vi "20191114_SR400 monitoring.vi"(10 "?":bool, 11 "?":bool) -> ()   [LabVIEW 2015]
uses:
  Libraries/SR400/Public/Typedefs/Counter.ctl
  Libraries/SR400/SR400.lvlib
panel:
  in  "Count Time Set":dbl[unit]=0.01
  in  "VISA resource name":refnum<visa-resource-name>="GPIB0::18::INSTR"
  out "Counts":dbl=46900.0 format="%#_6e"
  out "Count plot":dbl(graph)=46900.0
  # "Saturate @\n3E+7 c/s"
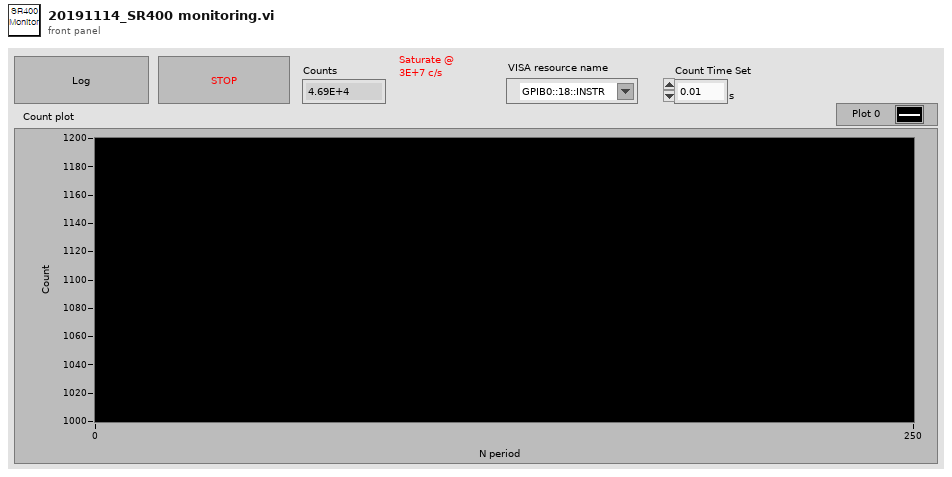
[diagram p1: front panel]
types:
  T1 = enum16{"open", "replace", "create", "open or create", "replace or create", "replace or create with confirmation"}
  T2 = typedef "SR400.lvlib/Counter.ctl" = enum16{"Counter A", "Counter B", "Counter T"}
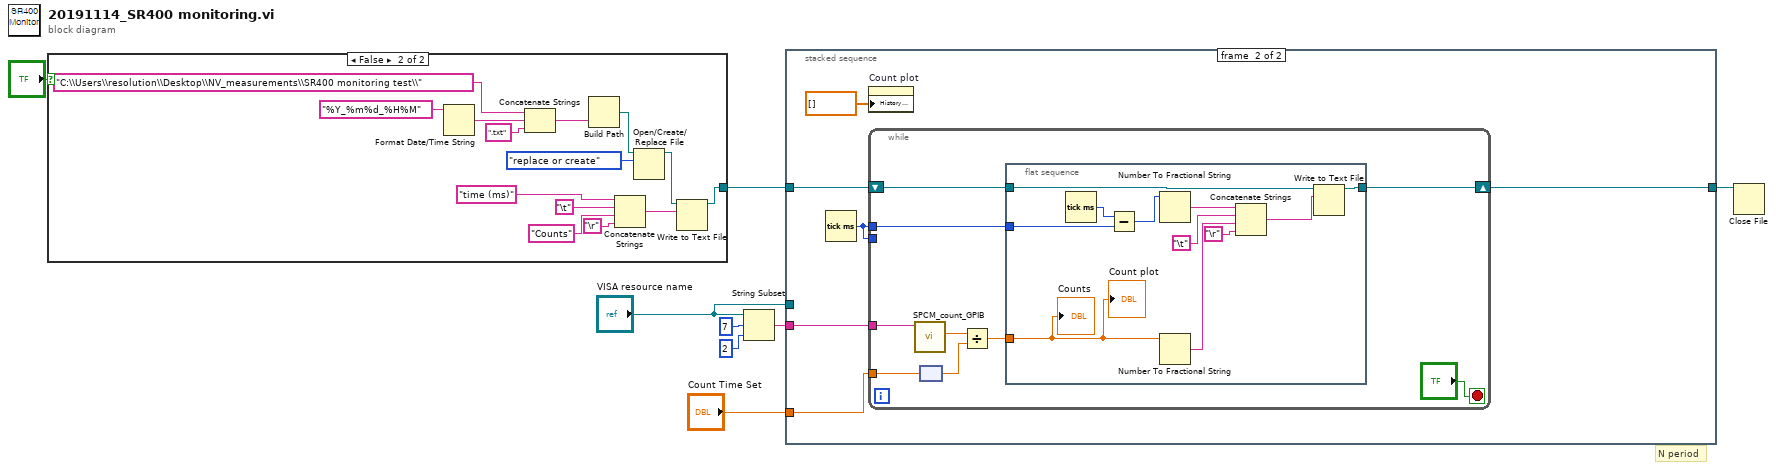
[diagram p0: block diagram]
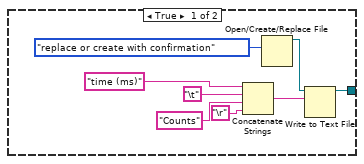
[diagram p2: hidden frame]
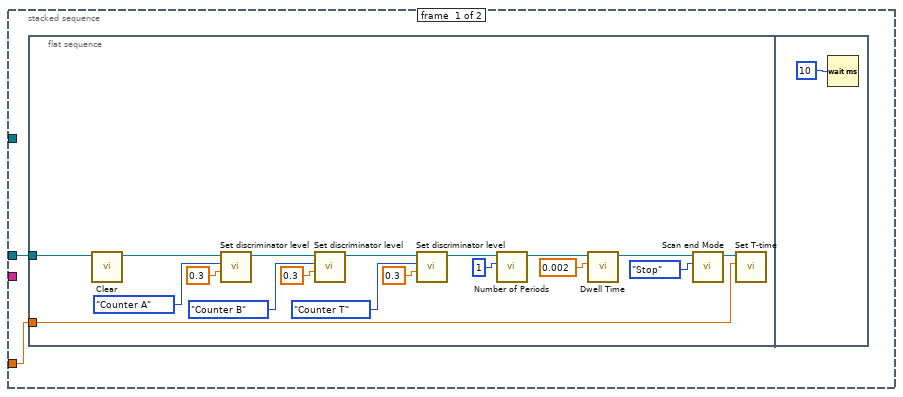
[diagram p3: hidden frame]
diagram:
  # "N period"
  n1 = case shown="False" "?" {
    tunnel: [w9 w22] -> w7
    frame True {
      n2 = Concatenate Strings("time (ms)" ("string"), "\t", "Counts" ("string"), "\r") -> (w15:string)
      n3 = Open/Create/Replace File(operation (0:open)=T1."replace or create with confirmation") -> (refnum out=w16:refnum<file>)  [unwired: 5 in, 2 out]
      n4 = Write to Text File(file (use dialog)=w16, text=w15) -> (refnum out=w9:refnum<file>)  [unwired: 2 in, 2 out]
    }
    frame False {
      n5 = Format Date/Time String(time format string (%c)="%Y_%m%d_%H%M") -> (date/time string=w27:string)  [unwired: 2 in]
      n6 = Concatenate Strings("C:\\Users\\resolution\\Desktop\\NV_measurements\\SR400 monitoring test\\" ("string"), w27, ".txt" ("string")) -> (w26:string)
      n7 = Build Path(name or relative path=w26) -> (appended path=w30:path)  [unwired: 1 in]
      n8 = Concatenate Strings("time (ms)" ("string"), "\t", "Counts" ("string"), "\r") -> (w17:string)
      n9 = Open/Create/Replace File(file path (use dialog)=w30, operation (0:open)=T1."replace or create") -> (refnum out=w23:refnum<file>)  [unwired: 4 in, 2 out]
      n10 = Write to Text File(file (use dialog)=w23, text=w17) -> (refnum out=w22:refnum<file>)  [unwired: 2 in, 2 out]
    }
  }
  n11 = String Subset(string="VISA resource name", offset (0)=7, length (rest)=2 ("length (rest)")) -> (substring=w2:string)
  n12 = stacked-sequence {
    tunnel: w2 -> [_ w57]
    tunnel: w7 -> [_ w55]
    tunnel: [_ w54] -> w6
    tunnel: "VISA resource name" -> [w32 _]
    tunnel: "Count Time Set" -> [w31 w52]
    frame #0 {
      n13 = flat-sequence {
        tunnel: w32 -> [w35]
        tunnel: w31 -> [w33]
        frame #0 {
          n14 = call "Clear.vi"("VISA resource name"=w35) -> ("VISA resource name out"=w50:refnum<visa-resource-name>)  [unwired: 9 in, 1 out]
          n15 = call "Set discriminator level.vi"("Level (-0.034 V)"=0.3, "Discriminator (def: A)"=Counter."Counter A", "VISA resource name"=w50) -> ("VISA resource name out"=w47:refnum<visa-resource-name>)  [unwired: 7 in, 1 out]
          n16 = call "Set discriminator level.vi"("Level (-0.034 V)"=0.3, "Discriminator (def: A)"=Counter."Counter B", "VISA resource name"=w47) -> ("VISA resource name out"=w44:refnum<visa-resource-name>)  [unwired: 7 in, 1 out]
          n17 = call "Set discriminator level.vi"("Level (-0.034 V)"=0.3, "Discriminator (def: A)"=Counter."Counter T", "VISA resource name"=w44) -> ("VISA resource name out"=w41:refnum<visa-resource-name>)  [unwired: 7 in, 1 out]
          n18 = call "Number of Periods.vi"("# of periods (def: 1)"=1, "VISA resource name"=w41) -> ("VISA resource name out"=w39:refnum<visa-resource-name>)  [unwired: 8 in, 1 out]
          n19 = call "Dwell Time.vi"("Dwell time (0.002 s)"=0.002, "VISA resource name"=w39) -> ("VISA resource name out"=w37:refnum<visa-resource-name>)  [unwired: 8 in, 1 out]
          n20 = call "Scan end Mode.vi"("Scan End Mode (Def: Stop)"=enum16{"Stop", "Start"}."Stop", "VISA resource name"=w37) -> ("VISA resource name out"=w34:refnum<visa-resource-name>)  [unwired: 8 in, 1 out]
          n21 = call "Set T-time.vi"("Count Time Set"=w33, "VISA resource name"=w34) -> ()  [unwired: 5 in, 3 out]
        }
        frame #1 {
          n22 = Wait (ms)(milliseconds to wait=u32 10) -> ()  [unwired: 1 out]
        }
      }
    }
    frame #1 {
      n23 = Tick Count (ms)() -> (millisecond timer value=w53:u32)
      n24 = property on="Count plot" class="WFChart (strict)"("History Data"=dbl[] []) -> ()  [unwired: 2 in, 2 out]
      n25 = while {
        tunnel: w57 -> [w66]
        tunnel: w53 -> [_]
        tunnel: w53 -> [w64]
        shift-right: [w63] -> w54
        shift-left: w55 -> [w65]
        tunnel: w52 -> [w60]
        stop <- "?" stop-if-true
        n26 = call "SPCM_count_GPIB.vi"("SR400 GPIB Address"=w66) -> ("Counts"=w61:dbl)  [unwired: 10 in]
        n27 = node(w60) -> (w59:dbl)
        n28 = Divide(x=w61, y=w59) -> (x/y=w58:dbl)
        n29 = flat-sequence {
          tunnel: w58 -> [w67]
          tunnel: w65 -> [w69]
          tunnel: w64 -> [w76]
          tunnel: [w68] -> w63
          frame #0 {
            n30 = Tick Count (ms)() -> (millisecond timer value=w77:u32)
            n31 = Subtract(x=w77, y=w76) -> (x-y=w73:u32)
            n32 = Number To Fractional String(number=w73) -> (F-format string=w72:string)  [unwired: 3 in]
            n33 = Number To Fractional String(number=w67) -> (F-format string=w71:string)  [unwired: 3 in]
            n34 = Concatenate Strings(w72, "\t", w71, "\r") -> (w70:string)
            n35 = Write to Text File(file (use dialog)=w69, text=w70) -> (refnum out=w68:refnum<file>)  [unwired: 2 in, 2 out]
            "Count plot" <- w67
            "Counts" <- w67
          }
        }
      }
    }
  }
  n36 = Close File(refnum=w6) -> ()  [unwired: 1 in, 2 out]
